vi "XOR 3.vi"(1 "z":bool, 2 "y 2":bool, 3 "x":bool) -> (0 "ok":bool)   [LabVIEW 2017]
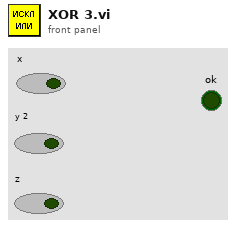
[diagram p1: front panel]
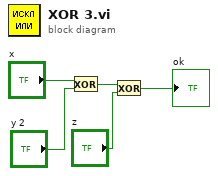
[diagram p0: block diagram]
diagram:
  n1 = Exclusive Or(1:"y 2", 2:"x") -> (0:w2:bool)
  n2 = Exclusive Or(1:"z", 2:w2) -> (0:→"ok":bool)
